vi "ConnectAsGRPC.vi"(8 "error in":errorcluster, 10 "Fully Qualified Name":string, 11 "Connection String":string) -> (0 "error out":errorcluster, 3 "MicronClient out":refnum<class "MicronClient.lvclass">)   [LabVIEW 2019, in "MicronGRPCClient.lvclass"]
uses:
  MicronGRPCClient.lvclass
  Base/Client/MicronClient.lvclass
  D:/GitHub/KarthikAbiram/Micron/LabVIEW/Source/vi.lib/Micron/Base/Client/MicronClient.lvclass
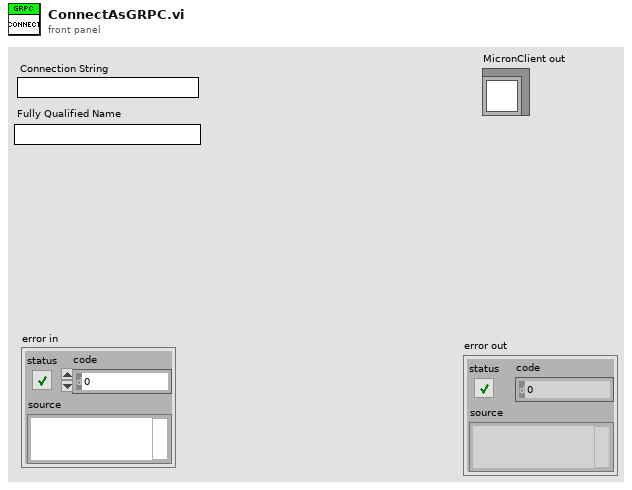
[diagram p1: front panel]
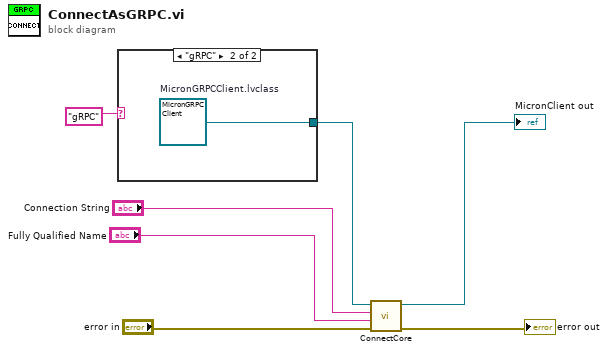
[diagram p0: block diagram]
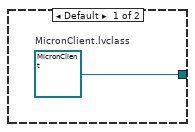
[diagram p2: hidden frame]
diagram:
  n1 = case shown="\"gRPC\"" "gRPC" {
    tunnel: [w8 w9] -> w5
    frame Default {
      w8 = refnum<class "MicronClient.lvclass"> refnum  # MicronClient.lvclass
    }
    frame "gRPC" {
      w9 = refnum<class "MicronGRPCClient.lvclass"> refnum  # MicronGRPCClient.lvclass
    }
  }
  n2 = call-dynamic "ConnectCore.vi"("error in (no error)"="error in", "Fully Qualified Name"="Fully Qualified Name", "Connection String"="Connection String", "MicronClient in"=w5) -> ("error out"=→"error out":errorcluster, "MicronClient out"=→"MicronClient out":refnum<class "MicronClient.lvclass">)  [unwired: 6 in]
